vi "PH_HamamatsuCamera.configure Cam.vi"(0 "VI in":refnum<vi>, 1 "Cam Handle in":i32, 2 "Parameter changed":bool, 3 "ROI changed":bool, 4 "Trigger Sets changed":bool, 5 "error in (no error)":errorcluster) -> (14 "VI out":refnum<vi>, 15 "Cam Handle out":i32, 18 "Cam Error out":errorcluster, 19 "error out":errorcluster)   [LabVIEW 2014, in "PH_HamamatsuCamera.lvlib"]
uses:
  PH_HamamatsuCamera.lvlib
  PH_HamamatsuCamera.Trigger Parameter.ctl
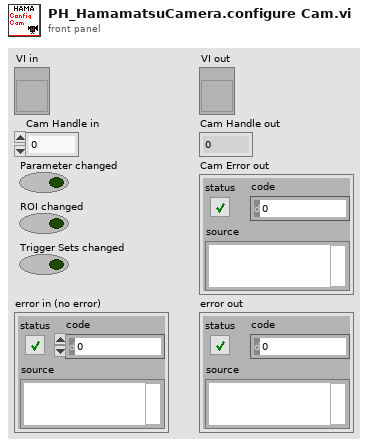
[diagram p1: front panel]
types:
  T1 = typedef "PH_HamamatsuCamera.lvlib/PH_HamamatsuCamera.Trigger Parameter.ctl" = cluster{"Mode":u32, "Polarity":u32, "Times":u32, "Delay":dbl}
  T2 = typedef "PH_HamamatsuCamera.lvlib/PH_HamamatsuCamera.i attribute.ctl" = cluster{"Gui Refs":cluster{"Camera Details":refnum<vi>, "ROI":refnum<vi>, "Set ROI to Maximum":refnum<vi>, "Trigger Parameters":refnum<vi>, "Brightness":refnum<vi>, "Shutter":refnum<vi>, "Gain":refnum<vi>, "Trigger Timeout":refnum<vi>, "Trigger Polarity":refnum<vi>, "Trigger Mode":refnum<vi>, "Parameters":refnum<vi>, "Set Cam Parameter":refnum<vi>, "Parameter to set":refnum<vi>, "Value to set":refnum<vi>}, "Cam":cluster{"Handle":i32, "Details":cluster{"Model":string, "Camera ID":string, "Firmware":string}, "Buffer Info":cluster{"height":u32, "width":u32, "datatype":u32}}, "H Offset":cluster{"Value":i32, "Minimum":i32, "Maximum":i32, "Increment":i32}, "V Offset":cluster{"Value":i32, "Minimum":i32, "Maximum":i32, "Increment":i32}, "H Width":cluster{"Value":i32, "Minimum":i32, "Maximum":i32, "Increment":i32}, "V Width":cluster{"Value":i32, "Minimum":i32, "Maximum":i32, "Increment":i32}, "Trigger Parameters":T1, "Trigger Timeout":u32, "Parameters":T3[], "Indicees Cam Parameters":cluster{"Brightness":i32, "Shutter":i32, "Gain":i32}, "Wanted Values":cluster{"Trigger Settings":T1[], "ROI":T4[], "Parameter":cluster{"Name":string, "Value":dbl}[]}}
  T3 = typedef "PH_HamamatsuCamera.lvlib/PH_HamamatsuCamera.Parameter Set.ctl" = cluster{"Parameter":string, "Value":dbl, "Writable":bool, "Range":cluster{"min":dbl, "max":dbl, "step":dbl}, "Default":dbl, "Value Names":cluster{"Name":string, "Value":dbl}[], "Text Values":bool}
  T4 = typedef "PH_HamamatsuCamera.lvlib/PH_HamamatsuCamera.ROI.ctl" = cluster{"Horizontal Offset":i32, "Vertical Offset":i32, "Horizontal Width":i32, "Vertical Width":i32}
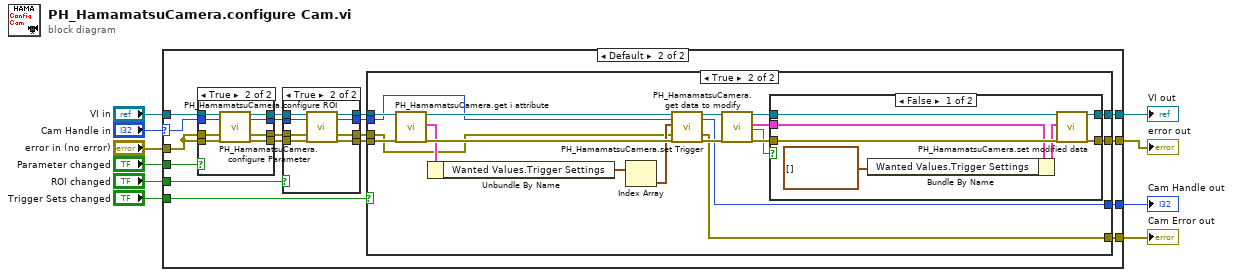
[diagram p0: block diagram]
diagram:
  n1 = case shown="Default" "Cam Handle in" {
    selector: "Cam Handle in" -> [w12 w25]
    tunnel: [w13 w28] -> w10
    tunnel: [w11 w27] -> w9
    tunnel: "VI in" -> [w13 w26]
    tunnel: "error in (no error)" -> [w11 w17]
    tunnel: [w12 w19] -> w8
    tunnel: [w11 w18] -> w7
    tunnel: "Parameter changed" -> [_ w16]
    tunnel: "ROI changed" -> [_ w15]
    tunnel: "Trigger Sets changed" -> [_ w14]
    frame -1 {
    }
    frame Default {
      n2 = case shown="True" w16 {
        tunnel: [w34 w43] -> w31
        tunnel: w26 -> [w35 w42]
        tunnel: w25 -> [w34 w41]
        tunnel: [w32 w40] -> w24
        tunnel: [w33 w39] -> w23
        tunnel: [w35 w38] -> w22
        tunnel: w17 -> [w33 w37]
        tunnel: w17 -> [w32 w36]
        frame False {
        }
        frame True {
          n3 = call "PH_HamamatsuCamera.configure Parameter.vi"("i ref in"=w42, "Cam Handle in"=w41, "Cam Error in"=w36, "error in (no error)"=w37) -> ("VI out"=w38:refnum<vi>, "Cam Handle out"=w43:i32, "Cam Error out"=w40:errorcluster, "error out"=w39:errorcluster)  [unwired: 12 in]
        }
      }
      n4 = case shown="True" w15 {
        tunnel: w31 -> [w78 w87]
        tunnel: [w76 w86] -> w30
        tunnel: [w79 w85] -> w29
        tunnel: w24 -> [w77 w84]
        tunnel: w23 -> [w76 w83]
        tunnel: w22 -> [w79 w82]
        tunnel: [w78 w81] -> w21
        tunnel: [w77 w80] -> w20
        frame False {
        }
        frame True {
          n5 = call "PH_HamamatsuCamera.configure ROI.vi"("VI in"=w82, "Cam Handle in"=w87, "Cam Error in"=w84, "error in (no error)"=w83) -> ("VI out"=w85:refnum<vi>, "Cam Handle out"=w81:i32, "Cam Error out"=w80:errorcluster, "error out"=w86:errorcluster)  [unwired: 12 in]
        }
      }
      n6 = case shown="True" w14 {
        tunnel: w30 -> [w45 w54]
        tunnel: w29 -> [w47 w56]
        tunnel: [w47 w59] -> w28
        tunnel: [w45 w62] -> w27
        tunnel: w21 -> [w46 w49]
        tunnel: w20 -> [w44 w48]
        tunnel: [w46 w65] -> w19
        tunnel: [w44 w64] -> w18
        frame False {
        }
        frame True {
          n7 = call "PH_HamamatsuCamera.get i attribute.vi"("i ref in"=w56, "error in (no error)"=w54) -> ("i ref out"=w55:refnum<vi>, "i attribute"=w52:T2, "error out"=w53:errorcluster)  [unwired: 15 in]
          n8 = Unbundle By Name(w52) -> ("Wanted Values.Trigger Settings"=w51:T1[])
          n9 = Index Array(array=w51) -> (element=w50:T1)  [unwired: 1 in]
          n10 = call "PH_HamamatsuCamera.set Trigger.vi"("i ref in"=w55, "Cam Handle in"=w49, "Trigger Parameters"=w50, "Cam Error in"=w48, "error in (no error)"=w53) -> ("i ref out"=w61:refnum<vi>, "Cam Handle out"=w65:i32, "Cam Error out"=w64:errorcluster, "error out"=w66:errorcluster)  [unwired: 11 in]
          n11 = call "PH_HamamatsuCamera.get data to modify.vi"("i ref in"=w61, "error in (no error)"=w66) -> ("i ref out"=w60:refnum<vi>, "i attribute"=w58:T2, "timed out"=w57:bool, "error out"=w63:errorcluster)  [unwired: 14 in]
          n12 = case shown="False" w57 {
            tunnel: w63 -> [w73 w74]
            tunnel: [w72 w74] -> w62
            tunnel: w60 -> [w71 w75]
            tunnel: [w70 w75] -> w59
            tunnel: w58 -> [w69 _]
            frame False {
              n13 = Bundle By Name(cluster=w69, "Wanted Values.Trigger Settings"=T1[] []) -> (w68:T2)
              n14 = call "PH_HamamatsuCamera.set modified data.vi"("i ref in"=w71, "i attribute"=w68, "error in (no error)"=w73) -> ("i ref out"=w70:refnum<vi>, "error out"=w72:errorcluster)  [unwired: 15 in]
            }
            frame True {
            }
          }
        }
      }
    }
  }
  "error out" <- w9
  "VI out" <- w10
  "Cam Handle out" <- w8
  "Cam Error out" <- w7
